vi "read.vi"(9 "connection ID":i32, 10 "bytes to read":i32=20, 11 "connection data":variant) -> (0 "error out":errorcluster)   [LabVIEW 2011]
uses:
  remaining_string.vi
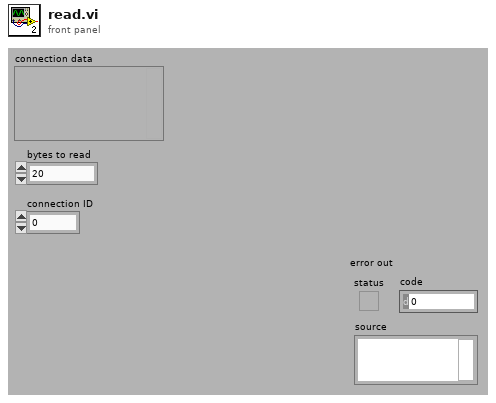
[diagram p1: front panel]
types:
  T1 = enum16{"Channel 1", "Channel 2", "Channel 3", "Real-Time Agent"}
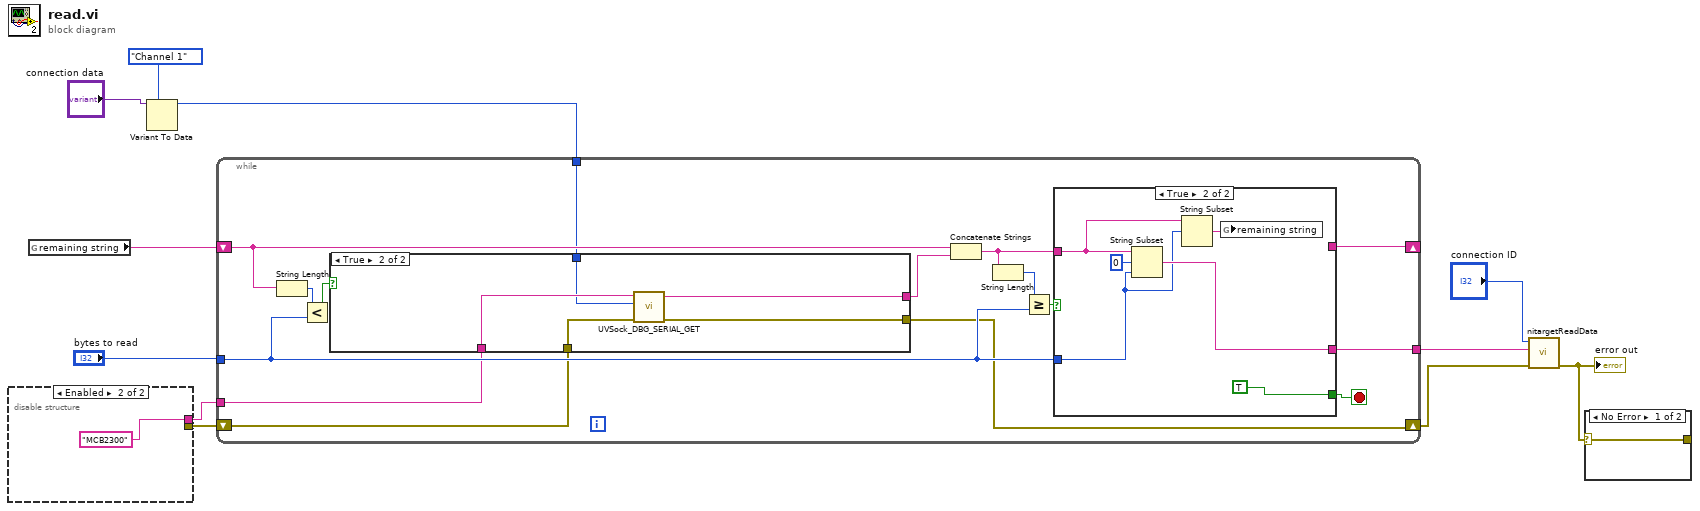
[diagram p0: block diagram]
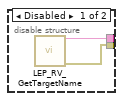
[diagram p3: hidden frame]
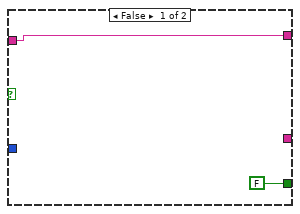
[diagram p5: hidden frame]
diagram:
  n1 = disable-structure shown="Enabled" {
    disable-tunnel: [w12 _] -> w3
    disable-tunnel: [w13 "MCB2300" ("Target Name")] -> w2
    frame Disabled {
      n2 = call "LEP_RV_GetTargetName.vi"() -> ("error out"=w12:errorcluster, "Target Name"=w13:string)  [unwired: 10 in]
    }
    frame Enabled {
    }
  }
  n3 = global read "remaining_string.vi" "remaining string"() -> (w4:string)
  n4 = Variant To Data(type=T1."Channel 1" ("Channel"), Variant="connection data") -> (data=w7:T1)  [unwired: 1 in, 1 out]
  n5 = while {
    shift-right: [w24] -> _
    shift-left: w4 -> [w22]
    tunnel: "bytes to read" -> [w20]
    tunnel: [w25] -> w11
    tunnel: w7 -> [w18]
    shift-right: [w17] -> w5
    shift-left: w3 -> [w16]
    tunnel: w2 -> [w15]
    stop <- w26 stop-if-true
    n6 = String Length(string=w22) -> (length=w21:i32)
    n7 = Less?(x=w21, y=w20) -> (x < y?=w19:bool)
    n8 = case shown="True" w19 {
      tunnel: [_ w35] -> w23
      tunnel: w18 -> [_ w31]
      tunnel: [w30 w34] -> w17
      tunnel: w16 -> [w30 w33]
      tunnel: w15 -> [_ w32]
      frame False {
      }
      frame True {
        n9 = call "UVSock_DBG_SERIAL_GET.vi"("error in (no error)"=w33, "Channel"=w31, "Target"=w32) -> ("error out"=w34:errorcluster, "Serial Data"=w35:string)  [unwired: 6 in, 1 out]
      }
    }
    n10 = Concatenate Strings(w22, w23) -> (w27:string)
    n11 = String Length(string=w27) -> (length=w29:i32)
    n12 = Greater Or Equal?(x=w29, y=w20) -> (x >= y?=w28:bool)
    n13 = case shown="True" w28 {
      tunnel: w27 -> [w37 w40]
      tunnel: w20 -> [_ w39]
      tunnel: [FALSE TRUE] -> w26
      tunnel: [_ w41] -> w25
      tunnel: [w37 _] -> w24
      frame False {
      }
      frame True {
        n14 = String Subset(string=w40, offset (0)=0, length (rest)=w39) -> (substring=w41:string)
        n15 = String Subset(string=w40, offset (0)=w39) -> (substring=w38:string)  [unwired: 1 in]
        n16 = global write "remaining_string.vi" "remaining string"(w38) -> ()
      }
    }
  }
  n17 = call <vilib>:"nitargetReadData.vi"("error in (no error)"=w5, "Data Read"=w11, "Connection ID"="connection ID") -> ("error out"=w1:errorcluster)  [unwired: 8 in]
  "error out" <- w1
  n18 = case shown="No Error" w1 {
    selector: w1 -> [w44 w45]
    tunnel: [w44 w45] -> _
    frame No Error {
    }
    frame Error {
    }
  }
